vi "判断vi是否在运行.vi"(3 "错误输入（无错误）":errorcluster, 5 "VI路径":path) -> (0 "错误输出":errorcluster, 1 "vi正在运行?":bool, 2 "引用输出":refnum<vi>)   [LabVIEW 2014]
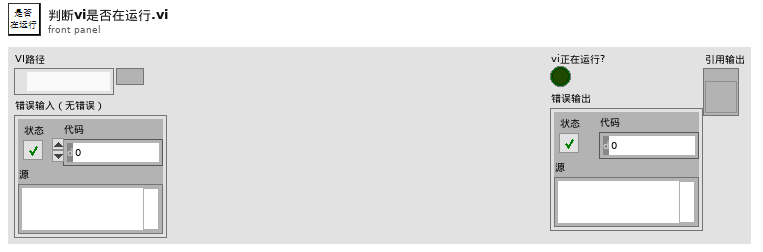
[diagram p1: front panel]
types:
  T1 = enum32{"Bad", "Idle", "Run top level", "Running"}
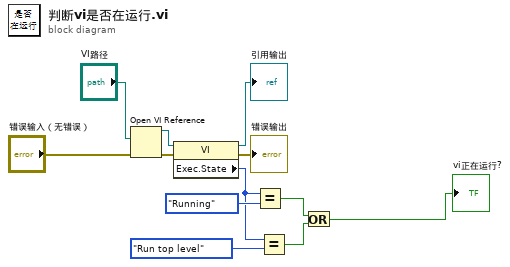
[diagram p0: block diagram]
diagram:
  n1 = Open VI Reference(vi path="VI路径", error in (no error)="错误输入（无错误）") -> (vi reference=w10:refnum<vi>, error out=w9:errorcluster)  [unwired: 4 in]
  n2 = property class="VI"(reference=w10, error in=w9) -> (reference out=→"引用输出":refnum<vi>, error out=→"错误输出":errorcluster, "Exec.State"=w4:T1)
  n3 = Equal?(x=w4, y=T1."Running" ("执行:状态")) -> (x = y?=w3:bool)
  n4 = Equal?(x=w4, y=T1."Run top level" ("执行:状态")) -> (x = y?=w2:bool)
  n5 = Or(x=w3, y=w2) -> (x .or. y?=→"vi正在运行?":bool)
